vi "Custom UUT Errors.vi"(8 "Error In":errorcluster, 11 "UUT Error File":path) -> (0 "Error Out":errorcluster)   [LabVIEW 2017, in "TSC Error.lvlib"]
doc: "Use this VI to set the path to a custom error file for a Unit Under Test (UUT).\n\nInputs:\n-UUT Error File [path] - the path to the UUT's custom error code definition file\n-error in\n\nOutputs:\n-error out\n__________________________________\n<b>Code Developed By:</b>\nDaniel Coons\nTechnology Service Corporation\n1983 S Liberty Drive\nBloomington, IN 47403\nPhone: 812 558-7100\ndaniel.coons@tsc.com\nwww.tsc.com\n\n<b>Date Created:</b> 04 APR 2016\n<b>Date Updated:</b>"
uses:
  TSC Error.lvlib
  _Messages/Error/Error.lvclass
  _Messages/ERROR_Add UUT Error/ERROR_Add UUT Error.lvclass
  C:/Development/Reuse-libraries/Error/_Messages/Error/Error.lvclass
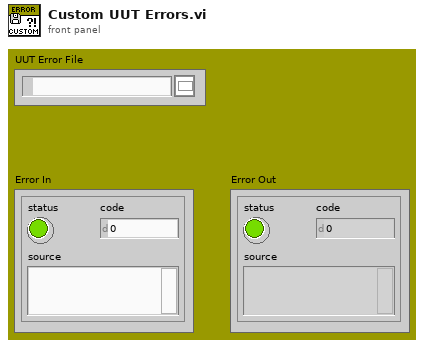
[diagram p1: front panel]
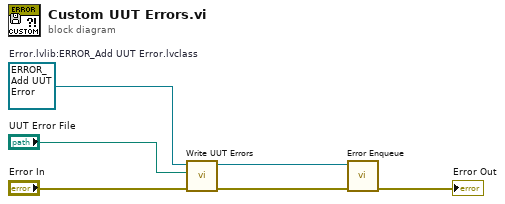
[diagram p0: block diagram]
diagram:
  w4 = refnum<class "ERROR_Add UUT Error.lvclass"> refnum  # Error.lvlib:ERROR_Add UUT Error.lvclass
  n1 = call "Write UUT Errors.vi"("error in (no error)"="Error In", "UUT Errors"="UUT Error File", "Error in"=w4) -> ("error out"=w2:errorcluster, "Error out"=w1:refnum<class "ERROR_Add UUT Error.lvclass">)  [unwired: 7 in]
  n2 = call "Error Enqueue.vi"("error in"=w2, "Error Message in"=w1) -> ("error out"=→"Error Out":errorcluster)  [unwired: 8 in, 1 out]
